vi "GetAvPowerE4418B.vi"(2 "Context":string, 4 "error in (no error)":errorcluster, 6 "IntervalBetweenReadings (mS)":i32=10 min=1 max=1000 step=1, 7 "N samples":i32=30 min=1 max=1000 step=1) -> (0 "Error out":errorcluster, 1 "VI dBSSD Power (dB)":dbl format="%#.10f", 3 "VI Mean Power (dBm)":dbl format="%#.10f", 5 "String_E4418A_Pwr":string)   [LabVIEW 2009]
doc: "Reads the power from the E4418B power meter."
uses:
  <vilib>/Analysis/NI_AALBase.lvlib
panel:
  out "Computed Power returned (dBm)":dbl format="%#.10f"
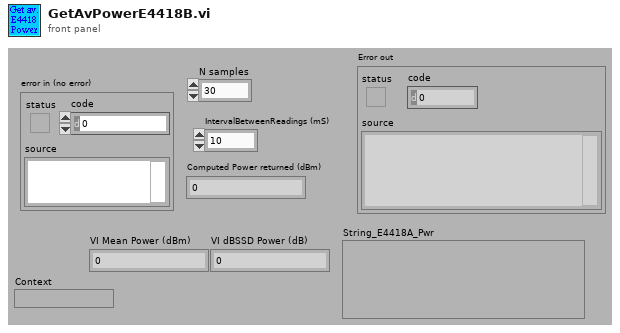
[diagram p1: front panel]
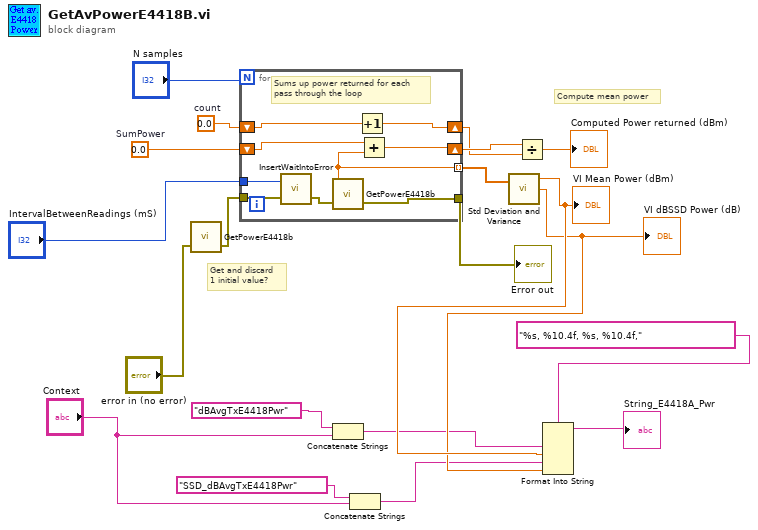
[diagram p0: block diagram]
diagram:
  w13 = 0.0  # count
  w20 = 0.0  # SumPower
  # "Get and discard\n1 initial value?"
  # "Compute mean power"
  n1 = call "GetPowerE4418b.vi"("error in (no error)"="error in (no error)") -> ("Error out"=w15:errorcluster)  [unwired: 1 in, 1 out]
  n2 = for {
    N: "N samples" -> [_]
    shift-right: [w28] -> w19
    shift-left: w20 -> [w29]
    tunnel: w15 -> [w23]
    tunnel: [w27] -> w16
    shift-right: [w25] -> w12
    shift-left: w13 -> [w26]
    tunnel: [w22] -> w11 mode=indexing
    tunnel: "IntervalBetweenReadings (mS)" -> [w21]
    # "Sums up power returned for each\npass through the loop"
    n3 = call "InsertWaitIntoError.vi"("error in (no error)"=w23, "Wait (msecs)"=w21) -> ("error out"=w24:errorcluster)  [unwired: 1 in]
    n4 = call "GetPowerE4418b.vi"("error in (no error)"=w24) -> ("Error out"=w27:errorcluster, "Power returned (dBm)"=w22:dbl)  [unwired: 1 in]
    n5 = Increment(x=w26) -> (x+1=w25:dbl)
    n6 = Add(x=w29, y=w22) -> (x+y=w28:dbl)
  }
  "Error out" <- w16
  n7 = Concatenate Strings("dBAvgTxE4418Pwr", "Context") -> (w5:string)
  n8 = Concatenate Strings("SSD_dBAvgTxE4418Pwr", "Context") -> (w4:string)
  n9 = call <vilib>:"Std Deviation and Variance.vi"("X"=w11) -> ("mean"=w9:dbl, "standard deviation"=w8:dbl)  [unwired: 1 in, 1 out]
  "VI Mean Power (dBm)" <- w9
  "VI dBSSD Power (dB)" <- w8
  n10 = Divide(x=w19, y=w12) -> (x/y=→"Computed Power returned (dBm)":dbl)
  n11 = Format Into String(format string="%s, %10.4f, %s, %10.4f,", w5, w9, w4, w8) -> (resulting string=→"String_E4418A_Pwr":string)  [unwired: 2 in, 1 out]
